vi "Botão Precess.vi"(0 "AR":string="6.014379870", 1 "Precessed Coord.":bool, 5 "Dec":string="-0.024612536", 7 "Temp local amb(K)":string="286.45", 9 "Pressao atm local (mB)":string="1014", 11 "Hum rel local":string=".50", 12 "Var RA":string="0", 13 "Var DEC":string="0") -> (4 "RA":dbl format="%.9f", 6 "DEC":dbl format="%.9f", 8 "Hora Sideral (rad)":dbl format="%.9f", 10 "Dist. Zenital (rad)":dbl format="%.9f", 14 "Observed HA (radians)":dbl, 15 "Massa de Ar":dbl format="%#.9f")   [LabVIEW 2018]
uses:
  Global_Telescopio.vi
panel:
  out "ativar botão GO":bool
  out "working area = VERDE":bool
  out "desativar botão GO":bool
  out "Piscar working area":bool
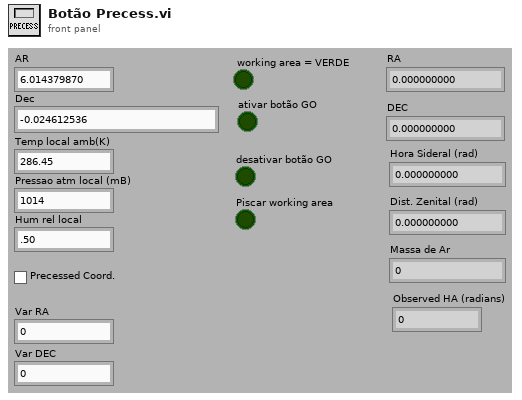
[diagram p1: front panel]
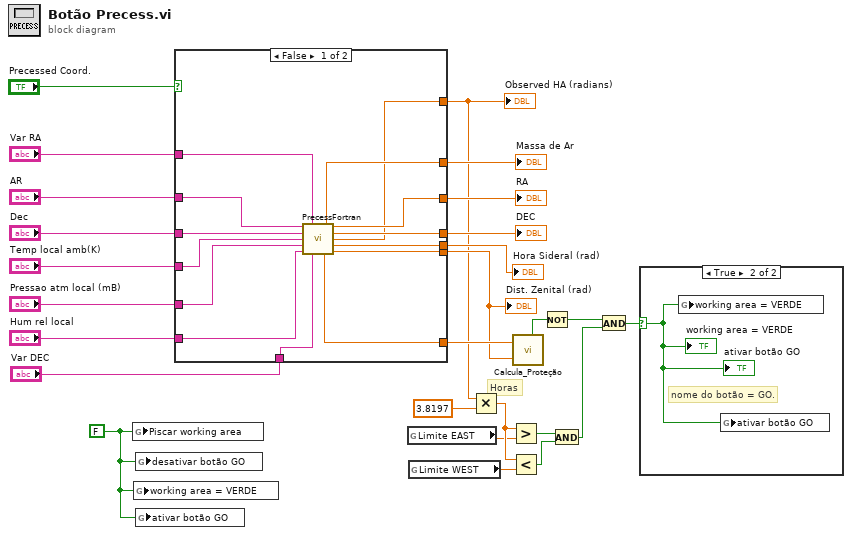
[diagram p0: block diagram]
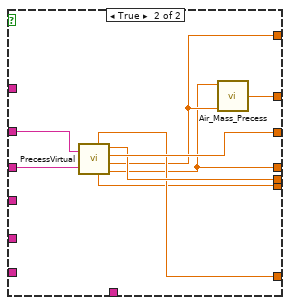
[diagram p2: hidden frame]
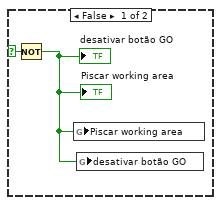
[diagram p3: hidden frame]
diagram:
  w26 = FALSE ("Piscar working area")
  # "Horas"
  n1 = global write "Global_Telescopio.vi" "Piscar working area"(w26) -> ()
  n2 = global write "Global_Telescopio.vi" "working area = VERDE"(w26) -> ()
  n3 = global write "Global_Telescopio.vi" "desativar botão GO"(w26) -> ()
  n4 = global write "Global_Telescopio.vi" "ativar botão GO"(w26) -> ()
  n5 = case shown="False" "Precessed Coord." {
    tunnel: "AR" -> [w40 w42]
    tunnel: "Dec" -> [w39 w41]
    tunnel: "Temp local amb(K)" -> [w38 _]
    tunnel: "Pressao atm local (mB)" -> [w37 _]
    tunnel: "Hum rel local" -> [w36 _]
    tunnel: [w35 w48] -> w20
    tunnel: [w34 w43] -> w19
    tunnel: [w33 w45] -> w11
    tunnel: [w32 w49] -> w18
    tunnel: [w31 w47] -> w17
    tunnel: "Var RA" -> [w30 _]
    tunnel: "Var DEC" -> [w29 _]
    tunnel: [w28 w44] -> w10
    tunnel: [w27 w46] -> w13
    frame False {
      n6 = call "PrecessFortran.vi"("Asc reta"=w40, "Var RA"=w30, "Declinação"=w39, "Temperatura (Kelvin)"=w38, "Pressao atmosferica (mB)"=w37, "Humidade relativa (0 a 1)"=w36, "Var DEC"=w29) -> ("Estimated air mass"=w32:dbl, "Observed RA (radians)"=w35:dbl, "Observed Dec (radians)"=w34:dbl, "Observed HA (radians)"=w28:dbl, "Local apparent sidereal time (radians)"=w31:dbl, "Observed Azimuth (radians: N=0,E=90)"=w27:dbl, "Observed Zenith Distance (radians)"=w33:dbl)  [unwired: 2 in]
    }
    frame True {
      n7 = call "PrecessVirtual.vi"("RA_texto_rad"=w42, "DEC_texto_rad"=w41) -> ("AZIMUTE"=w46:dbl, "ZENITAL ANGLE"=w45:dbl, "Sideral Time"=w47:dbl, "RA"=w48:dbl, "AH"=w44:dbl, "DEC"=w43:dbl)
      n8 = call "Air_Mass_Precess.vi"("delta"=w43, "AH"=w44) -> ("Air Mass"=w49:dbl)  [unwired: 5 in]
    }
  }
  "Dist. Zenital (rad)" <- w11
  "Massa de Ar" <- w18
  "DEC" <- w19
  "RA" <- w20
  "Hora Sideral (rad)" <- w17
  "Observed HA (radians)" <- w10
  n9 = global read "Global_Telescopio.vi" "Limite EAST"() -> (w3:dbl)
  n10 = global read "Global_Telescopio.vi" "Limite WEST"() -> (w4:dbl)
  n11 = Multiply(x=w10, y=3.8197) -> (x*y=w8:dbl)
  n12 = Greater?(x=w8, y=w3) -> (0:w7:bool)
  n13 = Less?(x=w8, y=w4) -> (x < y?=w2:bool)
  n14 = call "Calcula_Proteção.vi"("Zenital angle rad"=w11, "Azimute rad"=w13) -> ("Prot Zmax"=w12:bool)  [unwired: 4 out]
  n15 = Not(x=w12) -> (.not. x?=w5:bool)
  n16 = And(x=w7, y=w2) -> (x .and. y?=w1:bool)
  n17 = And(x=w5, y=w1) -> (x .and. y?=w6:bool)
  n18 = case shown="True" w6 {
    selector: w6 -> [w51 w52]
    frame False {
      n19 = Not(x=w51) -> (.not. x?=w50:bool)
      "Piscar working area" <- w50
      "desativar botão GO" <- w50
      n20 = global write "Global_Telescopio.vi" "Piscar working area"(w50) -> ()
      n21 = global write "Global_Telescopio.vi" "desativar botão GO"(w50) -> ()
    }
    frame True {
      # "nome do botão = GO."
      n22 = global write "Global_Telescopio.vi" "working area = VERDE"(w52) -> ()
      n23 = global write "Global_Telescopio.vi" "ativar botão GO"(w52) -> ()
      "working area = VERDE" <- w52
      "ativar botão GO" <- w52
    }
  }
